vi "RPI2 Enable SPI.vi"(8 "Error In":errorcluster, 11 "Install LV Data":T1={"SSH Session"=refnum, "Status Log"="", "Detailed Log"="", "Credentials"={"Hostname or IP"="192.168.7.2", "Username"="root", "Password"=""}, "Target Info"={"OS Version"="", "CPU"="", "Systemd Version"="", "Internet Access"=FALSE, "Device Type"="", "LV Installed Ver"="", "LV Available Ver"="", "LV Upgrade Available"=FALSE, "Hostname"="", "NIC Info"=[]}, "Reboot Required?"=FALSE}) -> (0 "Error Out":errorcluster, 1 "Log":string, 3 "Install LV Data":T1={"SSH Session"=refnum, "Status Log"="", "Detailed Log"="", "Credentials"={"Hostname or IP"="192.168.7.2", "Username"="root", "Password"=""}, "Target Info"={"OS Version"="", "CPU"="", "Systemd Version"="", "Internet Access"=FALSE, "Device Type"="", "LV Installed Ver"="", "LV Available Ver"="", "LV Upgrade Available"=FALSE, "Hostname"="", "NIC Info"=[]}, "Reboot Required?"=FALSE})   [LabVIEW 2014, in "LMH-LINX.lvlib"]
uses:
  <vilib>/MakerHub/LINX/LMH-LINX.lvlib
  <vilib>/MakerHub/LINX/Private/Utilties/Target Management/Install LV Data.ctl
  C:/Program Files (x86)/National Instruments/LabVIEW 2014/vi.lib/MakerHub/LINX/Resources/Renci.SshNet.dll
  Resources/Renci.SshNet.dll
  <vilib>/MakerHub/LINX/Private/Utilties/Target Management/Target Info.ctl
  <vilib>/MakerHub/LINX/Private/Utilties/Target Management/NIC Info.ctl
  <vilib>/MakerHub/LINX/Private/Utilties/Target Management/NIC Mode.ctl
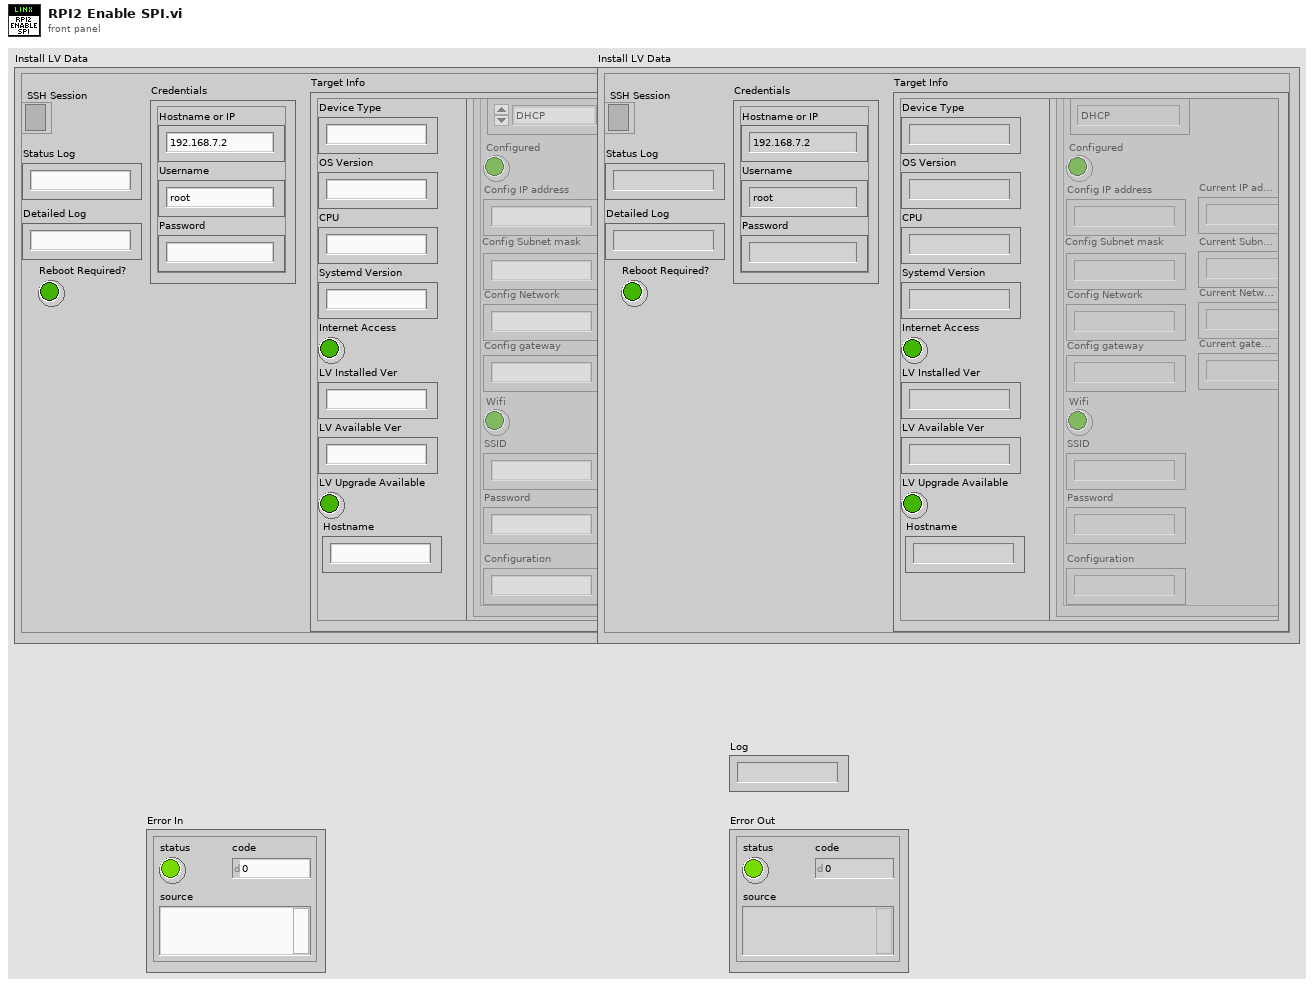
[diagram p1: front panel]
types:
  T1 = typedef "LMH-LINX.lvlib/Install LV Data.ctl" = cluster{"SSH Session":refnum<k24>, "Status Log":string, "Detailed Log":string, "Credentials":cluster{"Hostname or IP":string, "Username":string, "Password":string}, "Target Info":T2, "Reboot Required?":bool}
  T2 = typedef "LMH-LINX.lvlib/Target Info.ctl" = cluster{"OS Version":string, "CPU":string, "Systemd Version":string, "Internet Access":bool, "Device Type":string, "LV Installed Ver":string, "LV Available Ver":string, "LV Upgrade Available":bool, "Hostname":string, "NIC Info":T3[]}
  T3 = typedef "LMH-LINX.lvlib/NIC Info.ctl" = cluster{"Name":string, "NIC Mode":T4, "Configured":bool, "Config IP address":string, "Config Subnet mask":string, "Config Network":string, "Config gateway":string, "Wifi":bool, "SSID":string, "Password":string, "Configuration":string, "Current IP address":string, "Current Subnet mask":string, "Current gateway":string, "Current Network":string}
  T4 = typedef "LMH-LINX.lvlib/NIC Mode.ctl" = enum16{"DHCP", "Static", "Loopback"}
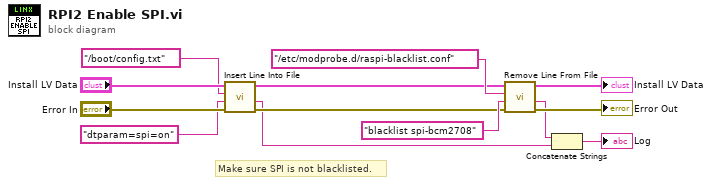
[diagram p0: block diagram]
diagram:
  # "Make sure SPI is not blacklisted."
  n1 = call <vilib>:"Insert Line Into File.vi"("Error In"="Error In", "Line"="dtparam=spi=on" ("File Path"), "File Path"="/boot/config.txt", "Install LV Data"="Install LV Data") -> ("Error Out"=w4:errorcluster, "Log"=w2:string, "Install LV Data"=w3:T1)  [unwired: 4 in, 1 out]
  n2 = call <vilib>:"Remove Line From File.vi"("Error In"=w4, "Line"="blacklist spi-bcm2708" ("File Path"), "File Path"="/etc/modprobe.d/raspi-blacklist.conf", "Install LV Data"=w3) -> ("Error Out"=→"Error Out":errorcluster, "Log"=w9:string, "Install LV Data"=→"Install LV Data":T1)  [unwired: 4 in, 1 out]
  n3 = Concatenate Strings(w9, w2) -> (→"Log":string)
